vi "Get_mean_array.vi"(1 "Moyenne_sur_?_pts 2":i32=5 min=1 step=2, 2 "InstFluxArray":sgl[](array[numeric])) -> (0 "Mean_Array":sgl[](array[numeric]))   [LabVIEW 2011]
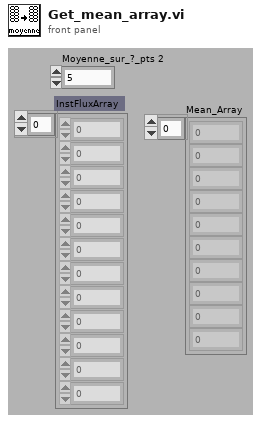
[diagram p1: front panel]
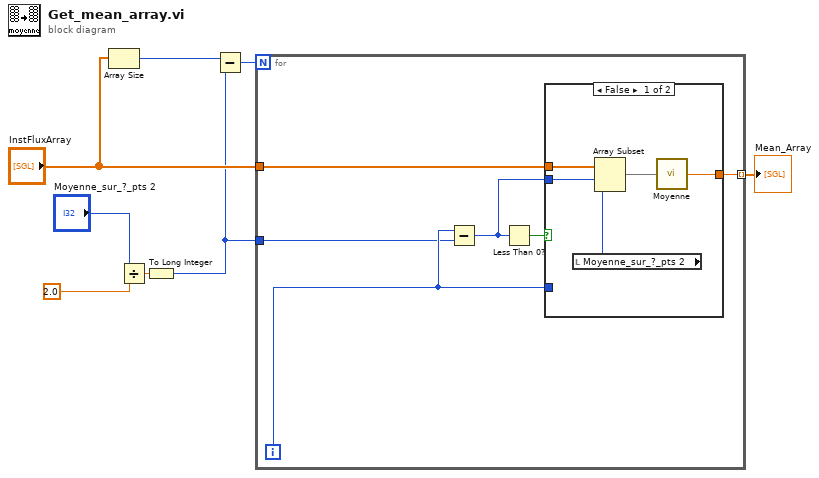
[diagram p0: block diagram]
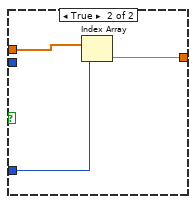
[diagram p2: hidden frame]
diagram:
  n1 = Array Size(array="InstFluxArray") -> (size(s)=w2:i32)
  n2 = Divide(x="Moyenne_sur_?_pts 2", y=2.0) -> (x/y=w6:dbl)
  n3 = To Long Integer(number=w6) -> (32bit integer=w1:i32)
  n4 = Subtract(x=w2, y=w1) -> (x-y=w3:i32)
  n5 = for {
    N: w3 -> [_]
    tunnel: "InstFluxArray" -> [w14]
    tunnel: [w13] -> w7 mode=indexing
    tunnel: w1 -> [w9]
    i -> [w11]
    n6 = Subtract(x=w11, y=w9) -> (x-y=w10:i32)
    n7 = Less Than 0?(x=w10) -> (x < 0?=w12:bool)
    n8 = case shown="False" w12 {
      tunnel: w14 -> [w19 w22]
      tunnel: [w17 w21] -> w13
      tunnel: w11 -> [_ w20]
      tunnel: w10 -> [w16 _]
      frame False {
        n9 = local read "Moyenne_sur_?_pts 2"() -> (w15:i32)
        n10 = Array Subset(array=w19, index=w16, length=w15) -> (w18:sgl[])
        n11 = call "Moyenne.vi"("DBL-Array"=w18) -> ("Moyenne"=w17:sgl)
      }
      frame True {
        n12 = Index Array(array=w22, index=w20) -> (element=w21:sgl)
      }
    }
  }
  "Mean_Array" <- w7
